vi "ParseLinkQuality.vi"(0 "offset":i32, 1 "data out":string) -> (2 "rssi":i8, 3 "timestamp":u32, 4 "LQI":i8, 5 "Bytes Read":i32)   [LabVIEW 2010]
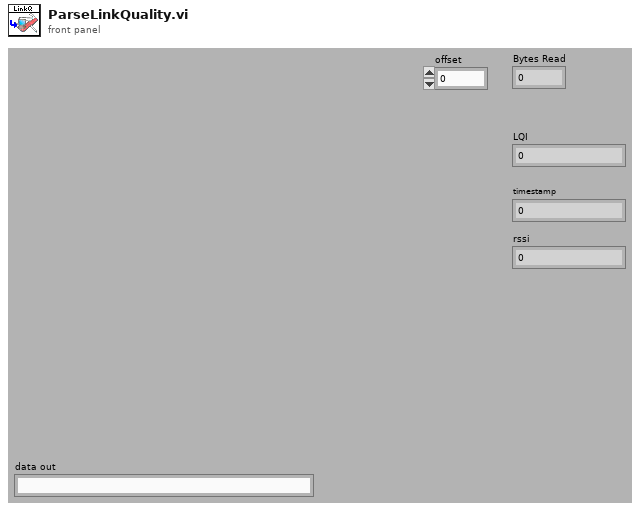
[diagram p1: front panel]
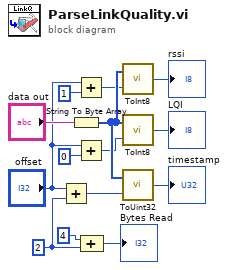
[diagram p0: block diagram]
diagram:
  w2 = 2 ("index")
  n1 = Add(x="offset", y=w2) -> (x+y=w3:i32)
  n2 = String To Byte Array(string="data out") -> (unsigned byte array=w8:u8[])
  n3 = Add(x="offset", y=1 ("index")) -> (x+y=w4:i32)
  n4 = Add(x="offset", y=0 ("index")) -> (x+y=w7:i32)
  n5 = Compound Arithmetic op=unknown(4 ("value"), w2) -> (→"Bytes Read":i32)
  n6 = call "ToInt8.vi"("index"=w4, "array"=w8) -> ("sp float"=→"rssi":i8)
  n7 = call "ToInt8.vi"("index"=w7, "array"=w8) -> ("sp float"=→"LQI":i8)
  n8 = call "ToUint32.vi"("index"=w3, "array"=w8) -> ("sp float"=→"timestamp":u32)
